vi "SampleCodeHowToFindRemovableDeviceChange.vi"() -> ()   [LabVIEW 2009]
uses:
  kernel32.dll
panel:
  out "Count":i32
  out "Drives Types":T1(array[ring])
  out "Drive Number":i32
  out "Drives":string[](array[string])
  in  "stop":bool
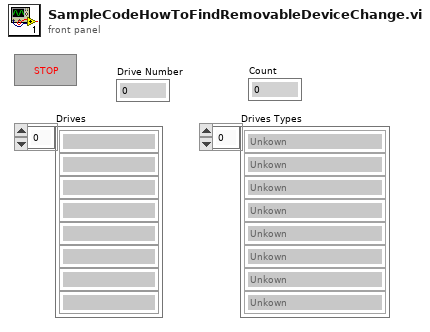
[diagram p1: front panel]
types:
  T1 = enum16{"Unkown", "No Root", "Removable", "Fixed", "Remote Drive", "CD Rom", "Ramdisk"}[]
  T2 = enum16{"Unkown", "No Root", "Removable", "Fixed", "Remote Drive", "CD Rom", "Ramdisk"}
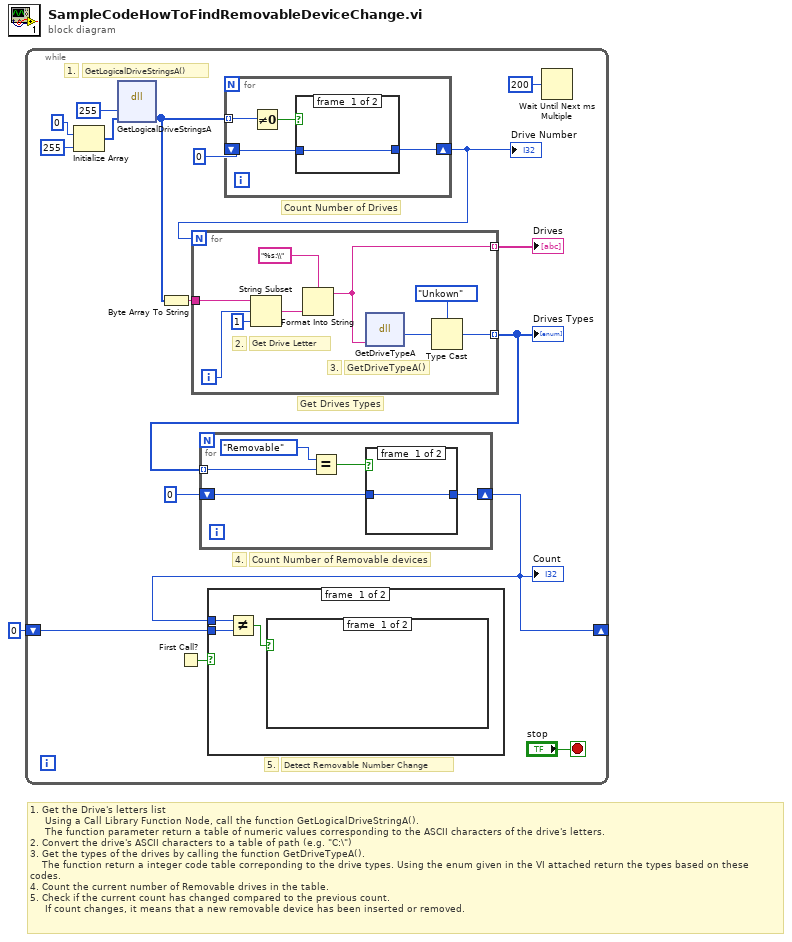
[diagram p0: block diagram]
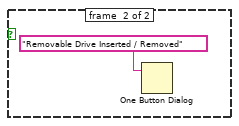
[diagram p2: hidden frame]
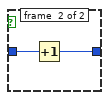
[diagram p4: hidden frame]
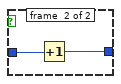
[diagram p5: hidden frame]
diagram:
  # "1. Get the Drive's letters list\n     Using a Call Library Function Node, call the function GetLogicalDriveStringA().\n     The function parameter return a table of numeric values corresponding to the ASCII characters of the drive's letters.\n2. Convert the drive's ASCII characters to a table of path (e.g. \"C:\\\")\n3. Get the types of the drives by calling the function GetDriveTypeA().\n    The function return a integer code table correponding to the drive types. Using the enum given in the VI attached return the types based on these codes.\n4. Count the current number of Removable drives in the table.\n5. Check if the current count has changed compared to the previous count.\n     If count changes, it means that a new removable device has been inserted or removed."
  n1 = while {
    shift-right: [w3] -> _
    shift-left: 0 -> [w4]
    stop <- "stop" stop-if-true
    # "5."
    # "4."
    # "1."
    # "Count Number of Drives"
    # "Get Drives Types"
    # "Count Number of Removable devices"
    # "Detect Removable Number Change"
    # "GetLogicalDriveStringsA()"
    n2 = Initialize Array(0 ("arg1"), 255 ("taille de la dimension")) -> (w14:i32[])
    n3 = dll-call lib="kernel32.dll" fn="GetLogicalDriveStringsA"("arg1"=255, "arg2"=w14) -> ("arg2"=w10:i32[])  [unwired: 4 in, 3 out]
    n4 = Byte Array To String(unsigned byte array=w10) -> (string=w8:string)
    n5 = First Call?() -> (First Call?: T/F=w5:bool)
    n6 = for {
      tunnel: w10 -> [w40] mode=indexing
      shift-right: [w41] -> w9
      shift-left: 0 -> [w42]
      n7 = Not Equal To 0?(x=w40) -> (x != 0?=w39:bool)
      n8 = case shown="True" w39 {
        tunnel: w42 -> [w43 w44]
        tunnel: [w43 w45] -> w41
        frame #0 {
        }
        frame #1 {
          n9 = Increment(x=w44) -> (x+1=w45:i32)
        }
      }
    }
    "Drive Number" <- w9
    n10 = for {
      N: w9 -> [_]
      tunnel: w8 -> [w35]
      tunnel: [w32] -> w7 mode=indexing
      tunnel: [w31] -> w2 mode=indexing
      i -> [w34]
      # "3."
      # "2."
      # "GetDriveTypeA()"
      # "Get Drive Letter"
      n11 = String Subset(string=w35, offset (0)=w34, length (rest)=1 ("longueur (reste)")) -> (substring=w36:string)
      n12 = Format Into String(format string="%s:\\", w36) -> (resulting string=w32:string)  [unwired: 2 in, 1 out]
      n13 = dll-call lib="kernel32.dll" fn="GetDriveTypeA"("lpRootPathName"=w32) -> ("type de retour"=w30:u16)  [unwired: 3 in, 3 out]
      n14 = Type Cast(type=T2."Unkown" ("Drive Type"), x=w30) -> (*(type *) &x=w31:T2)
    }
    "Drives" <- w7
    "Drives Types" <- w2
    n15 = for {
      tunnel: w2 -> [w26] mode=indexing
      shift-right: [w22] -> w3
      shift-left: 0 -> [w23]
      n16 = Equal?(x=T2."Removable" ("Drive Type"), y=w26) -> (x = y?=w24:bool)
      n17 = case shown="True" w24 {
        tunnel: w23 -> [w27 w29]
        tunnel: [w27 w28] -> w22
        frame #0 {
        }
        frame #1 {
          n18 = Increment(x=w29) -> (x+1=w28:i32)
        }
      }
    }
    "Count" <- w3
    n19 = case shown="False" w5 {
      tunnel: w4 -> [w19 _]
      tunnel: w3 -> [w20 _]
      frame #0 {
        n20 = Not Equal?(x=w20, y=w19) -> (x != y?=w18:bool)
        n21 = case shown="True" w18 {
          frame #0 {
          }
          frame #1 {
            n22 = One Button Dialog(message="Removable Drive Inserted / Removed") -> ()  [unwired: 2 out]
          }
        }
      }
      frame #1 {
      }
    }
    n23 = Wait Until Next ms Multiple(millisecond multiple=u32 200 ("n millisecondes")) -> ()  [unwired: 1 out]
  }
